vi "Update Plot Visible.vi"(8 "error in (no error)":errorcluster, 9 "Visible":bool, 10 "Index":i32, 11 "HistorianCharting in":refnum<class "HistorianCharting.lvclass">) -> (0 "error out":errorcluster, 3 "HistorianCharting out":refnum<class "HistorianCharting.lvclass">)   [LabVIEW 2020, in "VolatusGUIElements.lvlib" / "HistorianCharting.lvclass"]
uses:
  HistorianCharting.lvclass
  HistorianCharting.lvclass/HistorianCharting.ctl
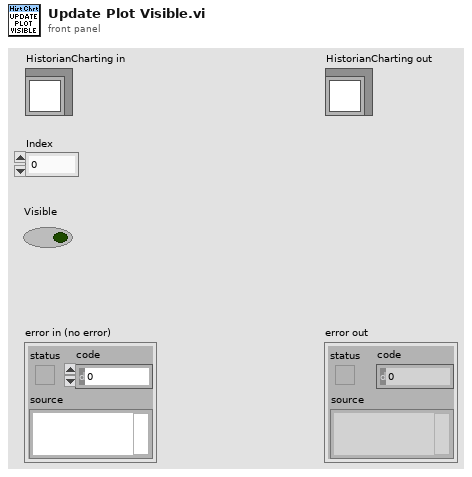
[diagram p1: front panel]
types:
  T1 = typedef "VolatusGUI.lvlib/Historian Charting Manager.lvclass/Plot Config.ctl" = cluster{"Channel":string, "Visible":bool, "Color":u32, "Scale":T2}
  T2 = typedef "VolatusGUI.lvlib/Historian Charting Manager.lvclass/Scale.ctl" = enum16{"Left", "Right"}
  T3 = typedef "VolatusGUI.lvlib/Historian Charting Manager.lvclass/Plot Group Config.ctl" = cluster{"Name":string, "X-Axis Type":T4, "X-Axis Channel":string, "Plots":T1[], "Lock Now":bool, "Time":string, "Swap Axes":bool}
  T4 = typedef "VolatusGUI.lvlib/Historian Charting Manager.lvclass/X-Axis Type.ctl" = enum16{"Time", "Channel"}
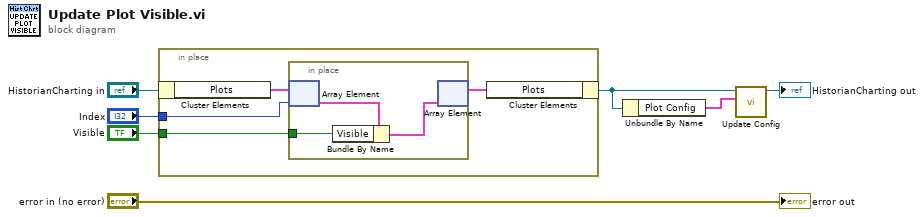
[diagram p0: block diagram]
diagram:
  n1 = in-place {
    in-place-border: "Index" -> [w10]
    in-place-border: "Visible" -> [w9]
    n2 = in-place-cluster #1("HistorianCharting in") -> ("Plots"=w11:T1[])
    n3 = in-place {
      in-place-border: w9 -> [w13]
      n4 = in-place-array #2(w11, w10) -> (w14:T1)
      n5 = Bundle By Name(cluster=w14, "Visible"=w13) -> (w12:T1)
      n6 = in-place-array #2(w12) -> (w8:T1[])  [unwired: 1 out]
    }
    n7 = in-place-cluster #1("Plots"=w8) -> (w5:refnum<class "HistorianCharting.lvclass">)
  }
  n8 = Unbundle By Name(w5) -> ("Plot Config"=w1:T3)
  n9 = call "Update Config.vi"("Config"=w1, "HistorianCharting in"=w5) -> ("HistorianCharting out"=→"HistorianCharting out":refnum<class "HistorianCharting.lvclass">)  [unwired: 8 in, 1 out]
  "error out" <- "error in (no error)"
